vi "Event-Timeout.vi"(8 "error in (no error)":errorcluster, 10 "Data ref. in":refnum<data-value>, 11 "UI ref. in":refnum<data-value>) -> (0 "error out":errorcluster, 2 "Data ref.":refnum<data-value>, 3 "UI ref.":refnum<data-value>)   [LabVIEW 2013, in "CameraVision.lvlib" / "CV-UI.lvclass"]
uses:
  CV-UI.lvclass
  Main/CV-Main.lvclass
  Main/Main-actions.ctl
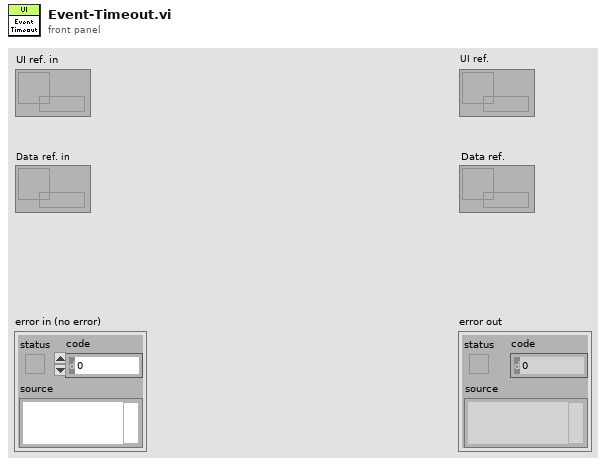
[diagram p1: front panel]
types:
  T1 = typedef "CameraVision.lvlib/CV-Main.lvclass/Main-actions.ctl" = enum16{"Idle", "Initialize", "Load defaults", "Update settings", "Check settings", "Save settings", "Save settings with dialog", "Load settings", "Load data", "Activate", "Start", "Wait for start signal", "Acquire & process", "Iterate", "Stop", "Refresh display", "Refresh status", "View camera settings", "View grabber settings", "Exit"}
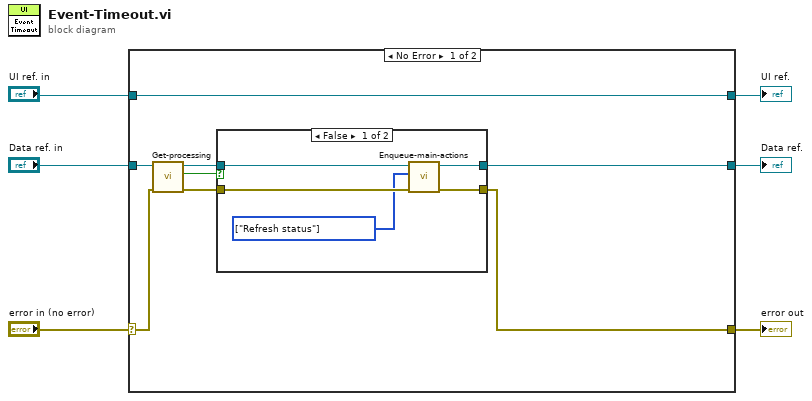
[diagram p0: block diagram]
diagram:
  n1 = case shown="No Error" "error in (no error)" {
    selector: "error in (no error)" -> [w11 w24]
    tunnel: [w7 w24] -> w5
    tunnel: [w14 w23] -> w3
    tunnel: "UI ref. in" -> [w14 w23]
    tunnel: "Data ref. in" -> [w13 w22]
    tunnel: [w8 w22] -> w1
    frame No Error {
      n2 = call "Get-processing.vi"("error in (no error)"=w11, "Data ref. in"=w13) -> ("error out"=w12:errorcluster, "Processing?"=w9:bool, "Data ref."=w10:refnum<data-value>)  [unwired: 7 in]
      n3 = case shown="False" w9 {
        tunnel: w12 -> [w19 w20]
        tunnel: [w17 w20] -> w7
        tunnel: w10 -> [w16 w21]
        tunnel: [w15 w21] -> w8
        frame False {
          w18 = T1[] [enum."Refresh status"] items=["Idle", "Initialize", "Load defaults", "Update settings", "Check settings", "Save settings", "Save settings with dialog", "Load settings", "Load data", "Activate", "Start", "Wait for start signal", "Acquire & process", "Iterate", "Stop", "Refresh display", "Refresh status", "View camera settings", "View grabber settings", "Exit"] ("State array")
          n4 = call "Enqueue-main-actions.vi"("error in (no error)"=w19, "State array"=w18, "Data ref. in"=w16) -> ("error out"=w17:errorcluster, "Data ref."=w15:refnum<data-value>)  [unwired: 6 in, 1 out]
        }
        frame True {
        }
      }
    }
    frame Error {
    }
  }
  "error out" <- w5
  "Data ref." <- w1
  "UI ref." <- w3
